vi "GetText.vi"(8 "error in":errorcluster, 11 "node in":refnum<class "Job Initialize.lvclass">) -> (0 "error out":errorcluster, 1 "additional text":string, 2 "text":string, 3 "node out":refnum<class "Job Initialize.lvclass">, 4 "glyph":string)   [LabVIEW 2014, in "Job Initialize.lvclass"]
doc: "Returns the text representation of the node used for the tree control."
uses:
  Job Initialize.lvclass
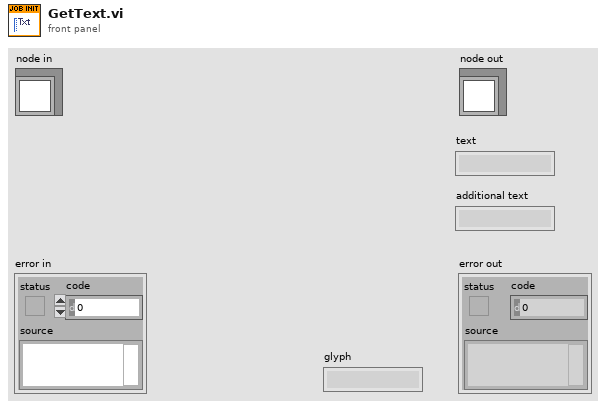
[diagram p1: front panel]
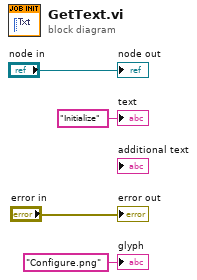
[diagram p0: block diagram]
diagram:
  "error out" <- "error in"
  "node out" <- "node in"
  "text" <- "Initialize" ("text")
  "glyph" <- "Configure.png" ("glyph")
